vi "Camera Image Server_Modified.vi"(10 "parameters":T1(array[cluster]), 11 "connection ID":refnum<k5>) -> ()   [LabVIEW 2017, in "VisionSystem.lvlib"]
uses:
  VisionSystem.lvlib
  <vilib>/Rock Robotics/SystemInterfaces/NetworkCommunication/NetComm_UsageReport_ResourceType.ctl
  TypeDefs/Cluster_Camera Settings.ctl
  <vilib>/Rock Robotics/WPI/Camera/WPI_CameraImageSize.ctl
  <vilib>/Rock Robotics/WPI/Camera/WPI_CameraFrameRate.ctl
  <vilib>/Rock Robotics/WPI/Camera/WPI_CameraWhite Balance Values.ctl
  <vilib>/Rock Robotics/WPI/Camera/WPI_CameraExposure Values.ctl
  Global_Vision Status.vi
  Global_Vision Server Data.vi
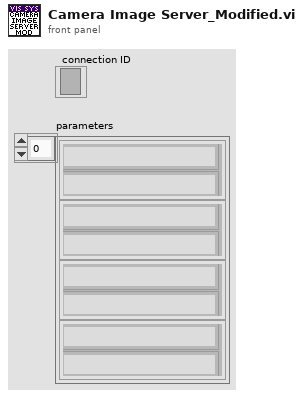
[diagram p1: front panel]
types:
  T1 = cluster{"token string":string, "token string 2":string}[]
  T2 = typedef "Cluster_Camera Settings.ctl" = cluster{"Image Size":T3, "Frame Rate (fps)":T4, "White Balance":T5, "Exposure":T6, "Exposure (%)":dbl, "Brightness":i32, "Sharpness":i32, "Saturation":i32}
  T3 = typedef "WPI_CameraImageSize.ctl" = enum16{"640x480", "320x240", "160x120", "Custom"}
  T4 = typedef "WPI_CameraFrameRate.ctl" = u32
  T5 = typedef "WPI_CameraWhite Balance Values.ctl" = enum16{"Auto", "Fixed indoor", "Fixed outdoor 1", "Fixed outdoor 2", "Fixed fluorescent 1", "Fixed fluorescent 2", "Hold current", "Custom"}
  T6 = typedef "WPI_CameraExposure Values.ctl" = enum16{"Auto", "Flicker-free 50 Hz", "Flicker-free 60 Hz", "Hold current", "Custom"}
  T7 = typedef "NetComm_UsageReport_ResourceType.ctl" = enum8{"Controller", "Module", "Language", "CANPlugin", "Accelerometer", "ADXL345", "AnalogChannel", "AnalogTrigger", "AnalogTriggerOutput", "CANJaguar", "Compressor", "Counter", "Dashboard", "DigitalInput", "DigitalOutput", "DriverStationCIO", "DriverStationEIO", "DriverStationLCD", "Encoder", "GearTooth", "Gyro", "I2C", "Framework", "Jaguar", "Joystick", "Kinect", "KinectStick", "PIDController", "Preferences", "PWM", "Relay", "RobotDrive", "SerialPort", "Servo", "Solenoid", "SPI", "Task", "Ultrasonic", "Victor", "Button", "Command", "AxisCamera", "PCVideoServer", "SmartDashboard", "Talon", "HiTechnicColorSensor", "HiTechnicAccel", "HiTechnicCompass", "SRF08", "AnalogOutput", "Victor SP", "Talon SRX", "CAN Talon SRX", "ADXL362 Accel", "ADXRS450 Gyro", "Rev SPARK", "Mindsensors SD540", "Digital Filter", "ADIS16448", "PDP", "PCM", "PigeonIMU", "Nidec Brushless", "CTRE CANifier", "CTRE Future 0", "CTRE Future 1", "CTRE Future 2", "CTRE Future 3", "CTRE Future 4", "CTRE Future 5", "CTRE Future 6"}
  T8 = enum16{"Update Mode", "Get Image", "Get Image Data"}
  T9 = typedef "IMAQ Image.ctl" = refnum<image>
  T10 = typedef "Image Type" = u32
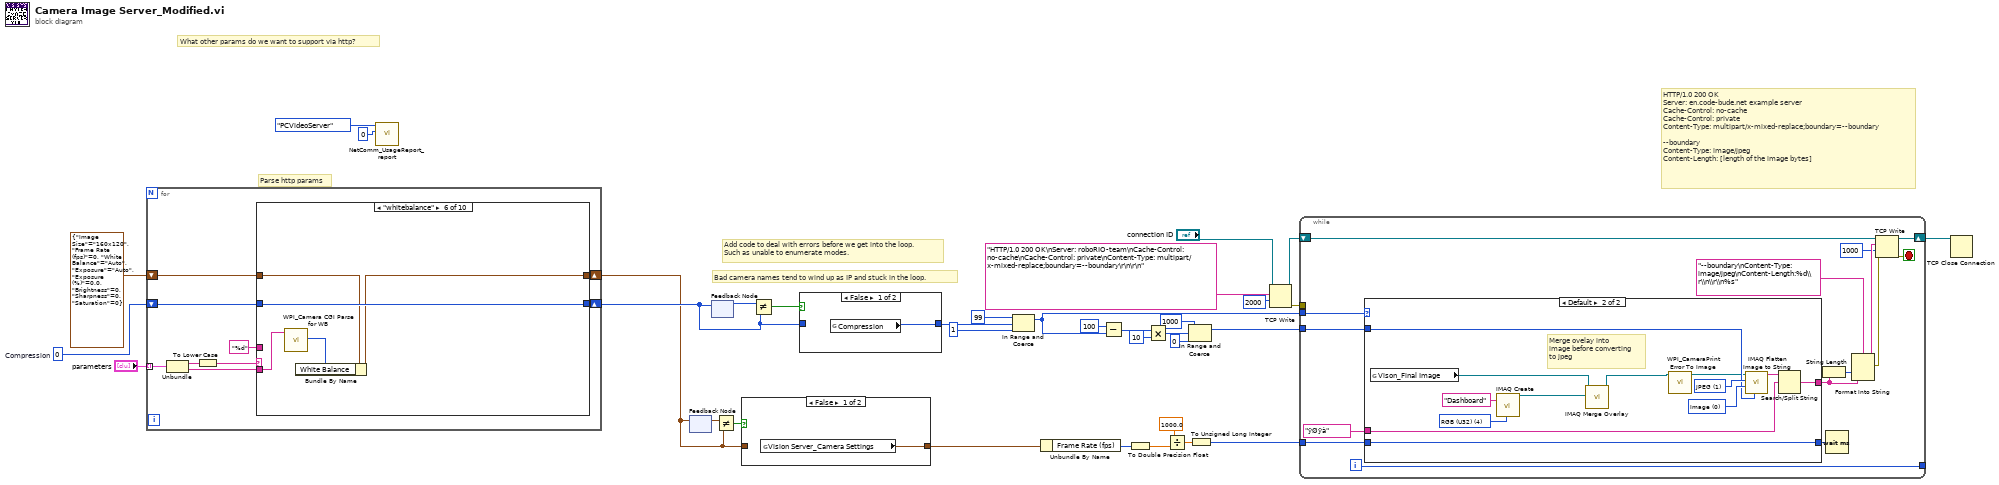
[diagram p0: block diagram]
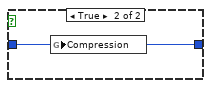
[diagram p2: hidden frame]
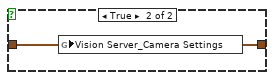
[diagram p3: hidden frame]
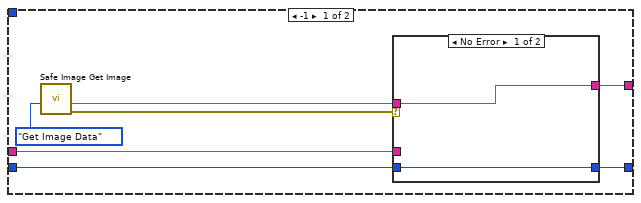
[diagram p4: hidden frame]
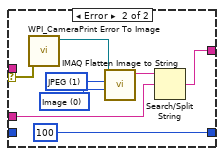
[diagram p5: hidden frame]
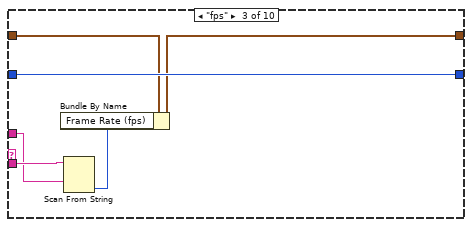
[diagram p8: hidden frame]
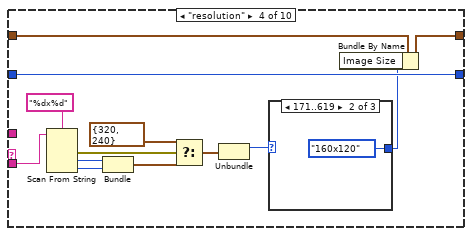
[diagram p9: hidden frame]
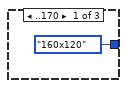
[diagram p10: hidden frame]
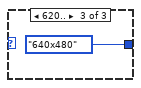
[diagram p11: hidden frame]
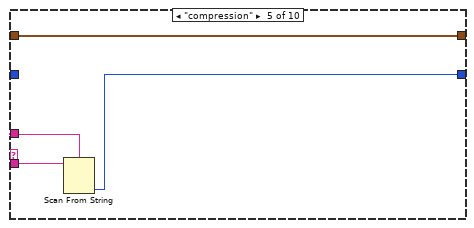
[diagram p12: hidden frame]
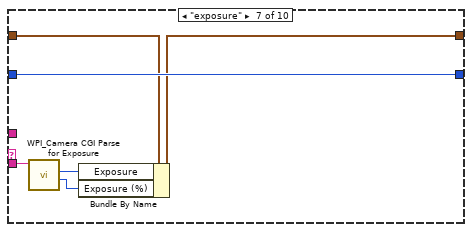
[diagram p13: hidden frame]
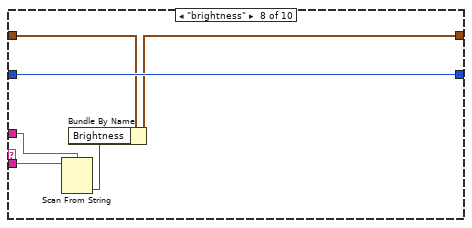
[diagram p14: hidden frame]
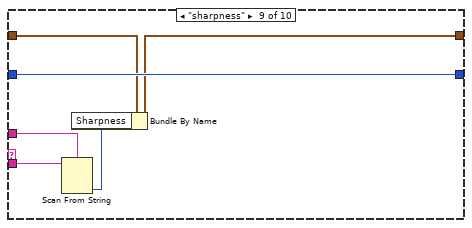
[diagram p15: hidden frame]
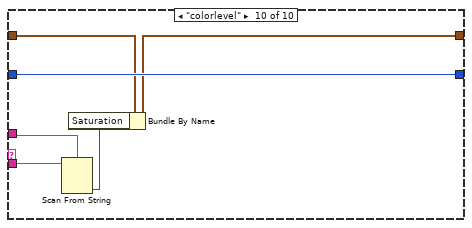
[diagram p16: hidden frame]
diagram:
  w9 = 0  # Compression
  # "Add code to deal with errors before we get into the loop.\nSuch as unable to enumerate modes."
  # "Parse http params"
  # "Bad camera names tend to wind up as IP and stuck in the loop."
  # "What other params do we want to support via http?"
  # "HTTP/1.0 200 OK\nServer: en.code-bude.net example server\nCache-Control: no-cache\nCache-Control: private\nContent-Type: multipart/x-mixed-replace;boundary=--boundary\n \n--boundary\nContent-Type: image/jpeg\nContent-Length: [length of the image bytes]"
  n1 = for {
    tunnel: "parameters" -> [w43] mode=indexing
    shift-right: [w37] -> w2
    shift-left: T2 {"Image Size"=enum."160x120", "Frame Rate (fps)"=0, "White Balance"=enum."Auto", "Exposure"=enum."Auto", "Exposure (%)"=0.0, "Brightness"=0, "Sharpness"=0, "Saturation"=0} ("Cam 0 Setings") -> [w38]
    shift-right: [w36] -> w4
    shift-left: w9 -> [w35]
    n2 = Unbundle(w43) -> ("token string"=w42:string, "token string 2"=w40:string)
    n3 = To Lower Case(string=w42) -> (all lower case string=w41:string)
    n4 = case shown="\"whitebalance\"" w41 {
      tunnel: w40 -> [_ _ w53 w57 w73 w75 w83 w89 w95 w101]
      tunnel: "%d" -> [_ _ w52 _ w72 _ _ w90 w96 w102]
      tunnel: w38 -> [w44 w46 w49 w65 w71 w77 w82 w86 w92 w98]
      tunnel: [w44 w46 w48 w64 w71 w76 w81 w85 w91 w97] -> w37
      tunnel: [w45 w47 w50 w66 w70 w78 w84 w87 w93 w99] -> w36
      tunnel: w35 -> [w45 w47 w50 w66 _ w78 w84 w87 w93 w99]
      frame Default {
      }
      frame "name" {
      }
      frame "fps" {
        n5 = Scan From String(format string=w52, input string=w53) -> (output 1=w51:i32)  [unwired: 3 in, 3 out]
        n6 = Bundle By Name(cluster=w49, "Frame Rate (fps)"=w51) -> (w48:T2)
      }
      frame "resolution" {
        n7 = Scan From String(format string="%dx%d", input string=w57) -> (error out=w61:errorcluster, output 1=w59:i32, output 2=w60:i32)  [unwired: 4 in, 2 out]
        n8 = Bundle(w59, w60) -> (w62:cluster{i32, i32})  [unwired: 1 in]
        n9 = Select(t=cluster{i32, i32} {320, 240} ("s? t:f"), s=w61, f=w62) -> (s? t:f=w56:cluster{i32, i32})
        n10 = Unbundle(w56) -> (w55:i32)  [unwired: 1 out]
        n11 = case shown="171..619" w55 {
          tunnel: [WPI_CameraImageSize."160x120" ("Image Size") WPI_CameraImageSize."160x120" ("Image Size") WPI_CameraImageSize."640x480" ("Image Size")] -> w54
          frame ..170 {
          }
          frame 171..619 {
          }
          frame 620.. {
          }
        }
        n12 = Bundle By Name(cluster=w65, "Image Size"=w54) -> (w64:T2)
      }
      frame "compression" {
        n13 = Scan From String(format string=w72, input string=w73) -> (output 1=w70:i32)  [unwired: 3 in, 3 out]
      }
      frame "whitebalance" {
        n14 = call <vilib>:"WPI_Camera CGI Parse for WB.vi"("String"=w75) -> ("enum"=w74:T5)  [unwired: 9 in, 1 out]
        n15 = Bundle By Name(cluster=w77, "White Balance"=w74) -> (w76:T2)
      }
      frame "exposure" {
        n16 = call <vilib>:"WPI_Camera CGI Parse for Exposure.vi"("String"=w83) -> ("Numeric"=w79:i32, "enum"=w80:T6)  [unwired: 9 in]
        n17 = Bundle By Name(cluster=w82, "Exposure"=w80, "Exposure (%)"=w79) -> (w81:T2)
      }
      frame "brightness" {
        n18 = Scan From String(format string=w90, input string=w89) -> (output 1=w88:i32)  [unwired: 3 in, 3 out]
        n19 = Bundle By Name(cluster=w86, "Brightness"=w88) -> (w85:T2)
      }
      frame "sharpness" {
        n20 = Scan From String(format string=w96, input string=w95) -> (output 1=w94:i32)  [unwired: 3 in, 3 out]
        n21 = Bundle By Name(cluster=w92, "Sharpness"=w94) -> (w91:T2)
      }
      frame "colorlevel" {
        n22 = Scan From String(format string=w102, input string=w101) -> (output 1=w100:i32)  [unwired: 3 in, 3 out]
        n23 = Bundle By Name(cluster=w98, "Saturation"=w100) -> (w97:T2)
      }
    }
  }
  n24 = call <vilib>:"NetComm_UsageReport_report.vi"("Instance Number"=u8 0, "Resource Type"=NetComm_UsageReport_ResourceType."PCVideoServer") -> ()  [unwired: 10 in]
  n25 = feedback-in #1(w2) -> ()
  n26 = feedback #1() -> (w8:T2)  [unwired: 1 in]
  n27 = feedback #2() -> (w6:i32)  [unwired: 1 in]
  n28 = feedback-in #2(w4) -> ()
  n29 = Not Equal?(x=w8, y=w2) -> (x != y?=w7:bool)
  n30 = case shown="False" w7 {
    tunnel: w2 -> [_ w104]
    tunnel: [w103 w104] -> w1
    frame False {
      n31 = global read "Global_Vision Server Data.vi" "Vision Server_Camera Settings"() -> (w103:T2)
    }
    frame True {
      n32 = global write "Global_Vision Server Data.vi" "Vision Server_Camera Settings"(w104) -> ()
    }
  }
  n33 = Not Equal?(x=w6, y=w4) -> (x != y?=w5:bool)
  n34 = case shown="False" w5 {
    tunnel: w4 -> [_ w106]
    tunnel: [w105 w106] -> w3
    frame False {
      n35 = global read "Global_Vision Server Data.vi" "Compression"() -> (w105:i32)
    }
    frame True {
      n36 = global write "Global_Vision Server Data.vi" "Compression"(w106) -> ()
    }
  }
  n37 = In Range and Coerce(upper limit=99, x=w3, lower limit=1) -> (coerced(x)=w11:i32)  [unwired: 1 out]
  n38 = Unbundle By Name(w1) -> ("Frame Rate (fps)"=w17:T4)
  n39 = Subtract(x=100, y=w11) -> (x-y=w23:i32)
  n40 = To Double Precision Float(number=w17) -> (double precision float=w19:dbl)
  n41 = Multiply(x=w23, y=10) -> (x*y=w25:i32)
  n42 = Divide(x=1000.0 ("port"), y=w19) -> (x/y=w28:dbl)
  n43 = In Range and Coerce(upper limit=1000, x=w25, lower limit=0) -> (coerced(x)=w21:i32)  [unwired: 1 out]
  n44 = To Unsigned Long Integer(number=w28) -> (unsigned 32bit integer=w18:u32)
  n45 = TCP Write(connection ID="connection ID", data in="HTTP/1.0 200 OK\nServer: roboRIO-team\nCache-Control: no-cache\nCache-Control: private\nContent-Type: multipart/x-mixed-replace;boundary=--boundary\r\n\r\n" ("regular expression"), 9:2000) -> (connection ID out=w16:refnum<k5>, error out=w15:errorcluster)  [unwired: 1 in, 1 out]
  n46 = while {
    shift-right: [w111] -> w34
    shift-left: w16 -> [w108]
    tunnel: w18 -> [w110]
    tunnel: w11 -> [w121]
    tunnel: w15 -> [_]
    tunnel: w21 -> [w120]
    tunnel: [w113] -> _
    i -> [w113]
    stop <- w112 stop-if-true
    n47 = case shown="Default" w121 {
      tunnel: [w126 w147] -> w117
      tunnel: w120 -> [_ w149]
      tunnel: "ÿØÿà" ("format string") -> [w125 w148]
      tunnel: w110 -> [w124 w144]
      tunnel: [w123 w144] -> w109
      frame -1 {
        n48 = call <vilib>:"Safe Image Get Image.vi"("Operation"=T8."Get Image Data") -> ("error out"=w128:errorcluster, "Image Data String"=w127:string)  [unwired: 7 in, 2 out]
        n49 = case shown="No Error" w128 {
          selector: w128 -> [_ w138]
          tunnel: [w130 w132] -> w126
          tunnel: w127 -> [w130 _]
          tunnel: w125 -> [_ w134]
          tunnel: w124 -> [w129 _]
          tunnel: [w129 u32 100 ("port")] -> w123
          frame No Error {
          }
          frame Error {
            w136 = 0 items=["Image", "Image and Vision Info", "Reference to Image"] ("Type of Flatten (Image and Vision Info)")
            w137 = 1 items=["None", "JPEG", "PACKED BINARY"] ("Compression (None)")
            n50 = call <vilib>:"WPI_CameraPrint Error To Image.vi"("error in (no error)"=w138) -> ("Image out"=w135:T9)  [unwired: 9 in, 1 out]
            n51 = call "IMAQ Flatten Image to String"("Type of Flatten (Image and Vision Info)"=w136, "Compression (None)"=w137, "Image"=w135) -> ("Data String"=w133:string)  [unwired: 7 in, 1 out]
            n52 = Search/Split String(string=w133, search string/char (-)=w134) -> (match + rest of string=w132:string)  [unwired: 1 in, 2 out]
          }
        }
      }
      frame Default {
        w142 = T10 4 items=["Grayscale (U8)", "Grayscale (I16)", "Grayscale (SGL)", "Complex (CSG)", "RGB (U32)", "HSL (U32)", "RGB (U64)", "Grayscale (U16)"] ("Image Type")
        w150 = 0 items=["Image", "Image and Vision Info", "Reference to Image"] ("Type of Flatten (Image and Vision Info)")
        w151 = 1 items=["None", "JPEG", "PACKED BINARY"] ("Compression (None)")
        # "Merge ovelay into\nimage before converting\nto jpeg"
        n53 = global read "Global_Vision Status.vi" "Vison_Final Image"() -> (w139:T9)
        n54 = call "IMAQ Create"("Image Name"="Dashboard", "Image Type"=w142) -> ("New Image"=w140:T9)  [unwired: 3 in, 1 out]
        n55 = call "IMAQ Merge Overlay"("Image Dst"=w140, "Image Src"=w139) -> ("Image Dst Out"=w141:T9)  [unwired: 8 in, 1 out]
        n56 = call <vilib>:"WPI_CameraPrint Error To Image.vi"("Image"=w141) -> ("Image out"=w145:T9)  [unwired: 9 in, 1 out]
        n57 = call "IMAQ Flatten Image to String"("Quality (750)"=w149, "Type of Flatten (Image and Vision Info)"=w150, "Compression (None)"=w151, "Image"=w145) -> ("Data String"=w146:string)  [unwired: 6 in, 1 out]
        n58 = Search/Split String(string=w146, search string/char (-)=w148) -> (match + rest of string=w147:string)  [unwired: 1 in, 2 out]
      }
    }
    n59 = String Length(string=w117) -> (length=w118:i32)
    n60 = Wait (ms)(milliseconds to wait=w109) -> ()  [unwired: 1 out]
    n61 = Format Into String(format string="--boundary\nContent-Type: image/jpeg\nContent-Length:%d\\r\\n\\r\\n%s" ("regular expression"), w118, w117) -> (resulting string=w115:string, error out=w116:errorcluster)  [unwired: 2 in]
    n62 = TCP Write(connection ID=w108, data in=w115, error in (no error)=w116, 9:1000 ("timeout ms (25000)")) -> (connection ID out=w111:refnum<k5>, error out=w112:errorcluster)  [unwired: 1 out]
  }
  n63 = TCP Close Connection(connection ID=w34) -> ()  [unwired: 1 in, 3 out]
